vi "Illini Hyperloop GUI v3.1.vi"() -> ()   [LabVIEW 2015]
uses:
  <vilib>/robotics/Controls/Attitude Indicator/Attitude Indicator.xctl
  CommunicationStatus.ctl
  StageEnum.ctl
  BlockDiagramControlEnum.ctl
  <vilib>/ErrorRing/Error Ring.xnode
panel:
  out "Braking Force":dbl
  out "Braking Force Chart":dbl(slide) caption="Braking Force (N)" scale=0.0..10000.0
  out "Current 6":dbl[unit] caption="Current"
  out "Voltage 6":dbl[unit] caption="Voltage"
  out "RPM 6":dbl[unit] caption="RPM"
  out "Current 5":dbl[unit] caption="Current"
  out "Voltage 5":dbl[unit] caption="Voltage"
  out "RPM 5":dbl[unit] caption="RPM"
  out "Current 4":dbl[unit] caption="Current"
  out "Voltage 4":dbl[unit] caption="Voltage"
  out "RPM 4":dbl[unit] caption="RPM"
  out "Current 3":dbl[unit] caption="Current"
  out "Voltage 3":dbl[unit] caption="Voltage"
  out "RPM 3":dbl[unit] caption="RPM"
  out "Current 2":dbl[unit] caption="Current"
  out "Voltage 2":dbl[unit] caption="Voltage"
  out "RPM 2":dbl[unit] caption="RPM"
  out "Current 1":dbl[unit] caption="Current"
  out "Voltage 1":dbl[unit] caption="Voltage"
  out "RPM 1":dbl[unit] caption="RPM"
  out "Flight Time":string
  out "Attitude Indicator":cluster{"Roll":dbl, "Pitch":dbl}(xcontrol)
  out "Yaw":dbl(knob) scale=-20.0..20.0
  out "RPM Gauge 6":dbl(knob) scale=0.0..2000.0
  out "RPM Gauge 5":dbl(knob) scale=0.0..2000.0
  out "RPM Gauge 4":dbl(knob) scale=0.0..2000.0
  out "RPM Gauge 3":dbl(knob) scale=0.0..2000.0
  out "RPM Gauge 2":dbl(knob) scale=0.0..2000.0
  out "RPM Gauge 1":dbl(knob) scale=0.0..2000.0
  out "Cabin Pressure":dbl format="%#.3g"
  out "Cabin Pressure (psi)":dbl(graph)
  out "Stage":T1
  out "Communication Status":T2
  out "Levitation Height":dbl[unit]
  out "Computing:":dbl format="%#.2g"
  out "Low Battery":dbl format="%#.2g"
  out "High Battery:":dbl format="%#.2g"
  out "Battery 3":dbl(slide) scale=0.0..100.0
  out "Battery 2":dbl(slide) scale=0.0..100.0
  out "Battery 1":dbl(slide) scale=0.0..100.0
  out "Z acceleration":dbl
  out "Y acceleration":dbl
  out "X acceleration":dbl
  out "Z velocity":dbl
  out "Y velocity":dbl
  out "X velocity":dbl
  out "Z position":dbl
  out "Y position":dbl
  out "X position":dbl
  out "Position (m)":dbl(slide) scale=0.0..2490.0
  out "Checkmark":u16(ring)
  out "Velocity (m/s)":dbl(graph)
  in  "EMERGENCY BRAKE":bool
  in  "Functional Test Tab Control":T3(tab)
  out "Functional Test A Data":string caption="Data:"
  in  "Functional Test 1":bool caption="Boolean"
  out "Functional Test B Data":string caption="Data:"
  in  "Functional Test 2":bool caption="Boolean"
  out "Functional Test C Data":string caption="Data:"
  in  "Functional Test 3":bool caption="Boolean"
  in  "Functional Test 4":bool caption="Boolean"
  out "Functional Test D Data":string caption="Data:"
  in  "Client Closed":string="The client VI closed the connection."
  out "Data out":string
  out "remote address":string
  out "remote port":u16
  in  "Prepare for Launch":bool caption="Boolean"
  in  "Stop Program":bool
  out "Temp 2:":dbl format="%.2g"
  out "Temp 1:":dbl format="%.2g"
  out "Temperature (K)":dbl[](graph)
  out "Acceleration Chart":dbl(graph)
  # "Illini Hyperloop"
  # "Arx Pax"
  # "Front"
  # "Attitude"
  # "Acceleration (m/s/s)"
  # "Battery Levels (%)"
  # "More battery?????"
  # "Functional Test A: Power Up and Communication"
  # "Functional Test B: Levitation"
  # "Functional Test C: Communication Inside Tube"
  # "Functional Test D: Internal power and Levitation"
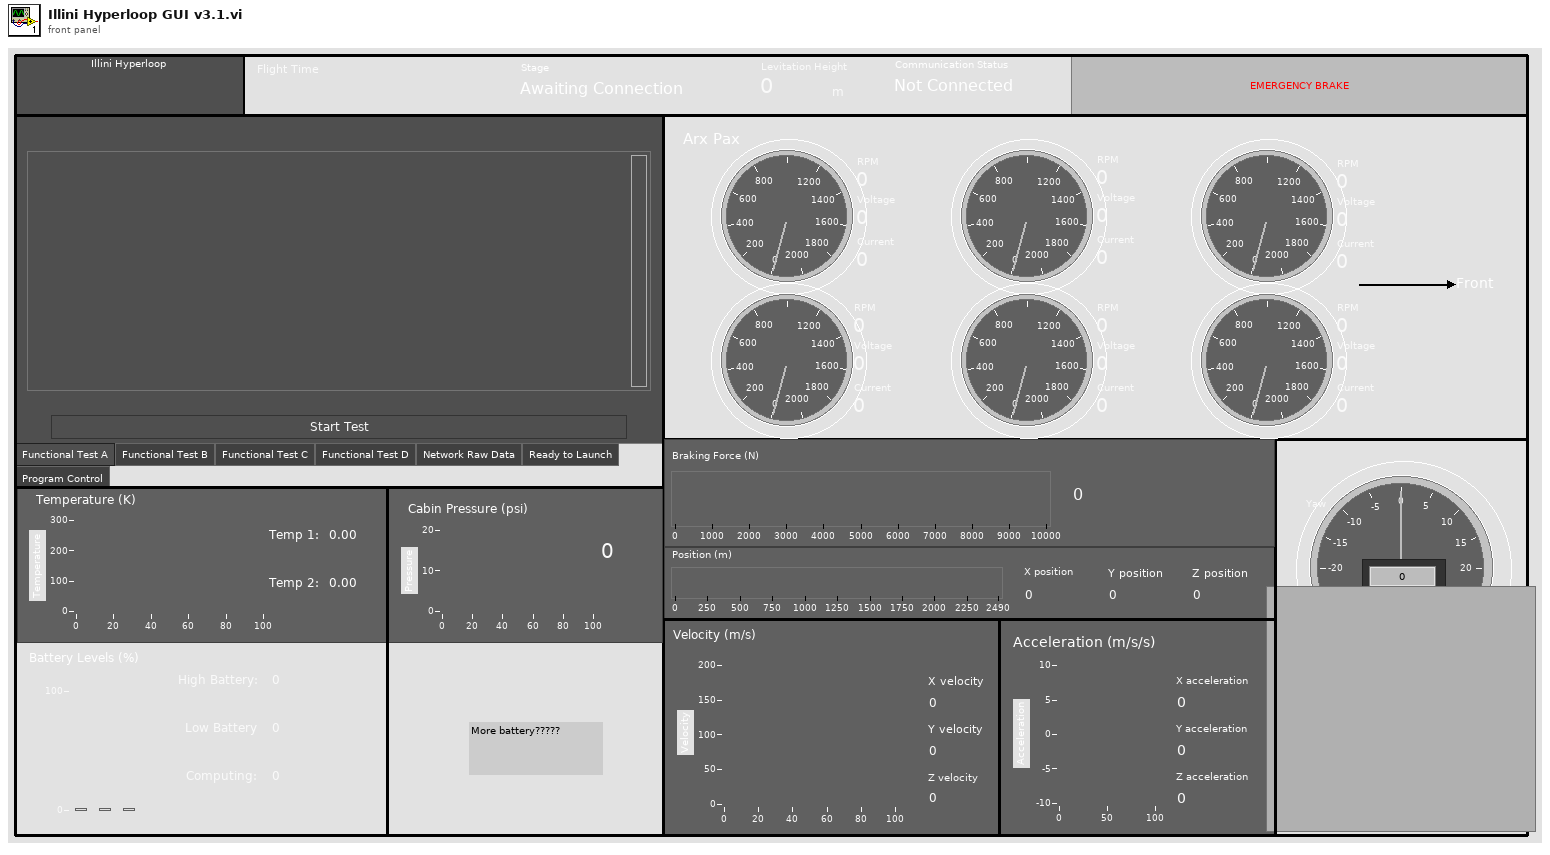
[diagram p1: front panel]
types:
  T1 = typedef "StageEnum.ctl" = enum16{"Awaiting Connection", "TEST Comms", "TEST Lev", "TEST Inside Comms", "TEST Internal Power", "Ready to Launch", "Acceleration", "Coast", "Brake"}
  T2 = typedef "CommunicationStatus.ctl" = enum16{"Not Connected", "Connected", "Disconnected"}
  T3 = enum32{"Functional Test A", "Functional Test B", "Functional Test C", "Functional Test D", "Network Raw Data", "Ready to Launch", "Program Control"}
  T4 = typedef "BlockDiagramControlEnum.ctl" = enum16{"Not Connected", "Disconnected", "Functional Test A", "Functional Test B", "Functional Test C", "Functional Test D", "Flight"}
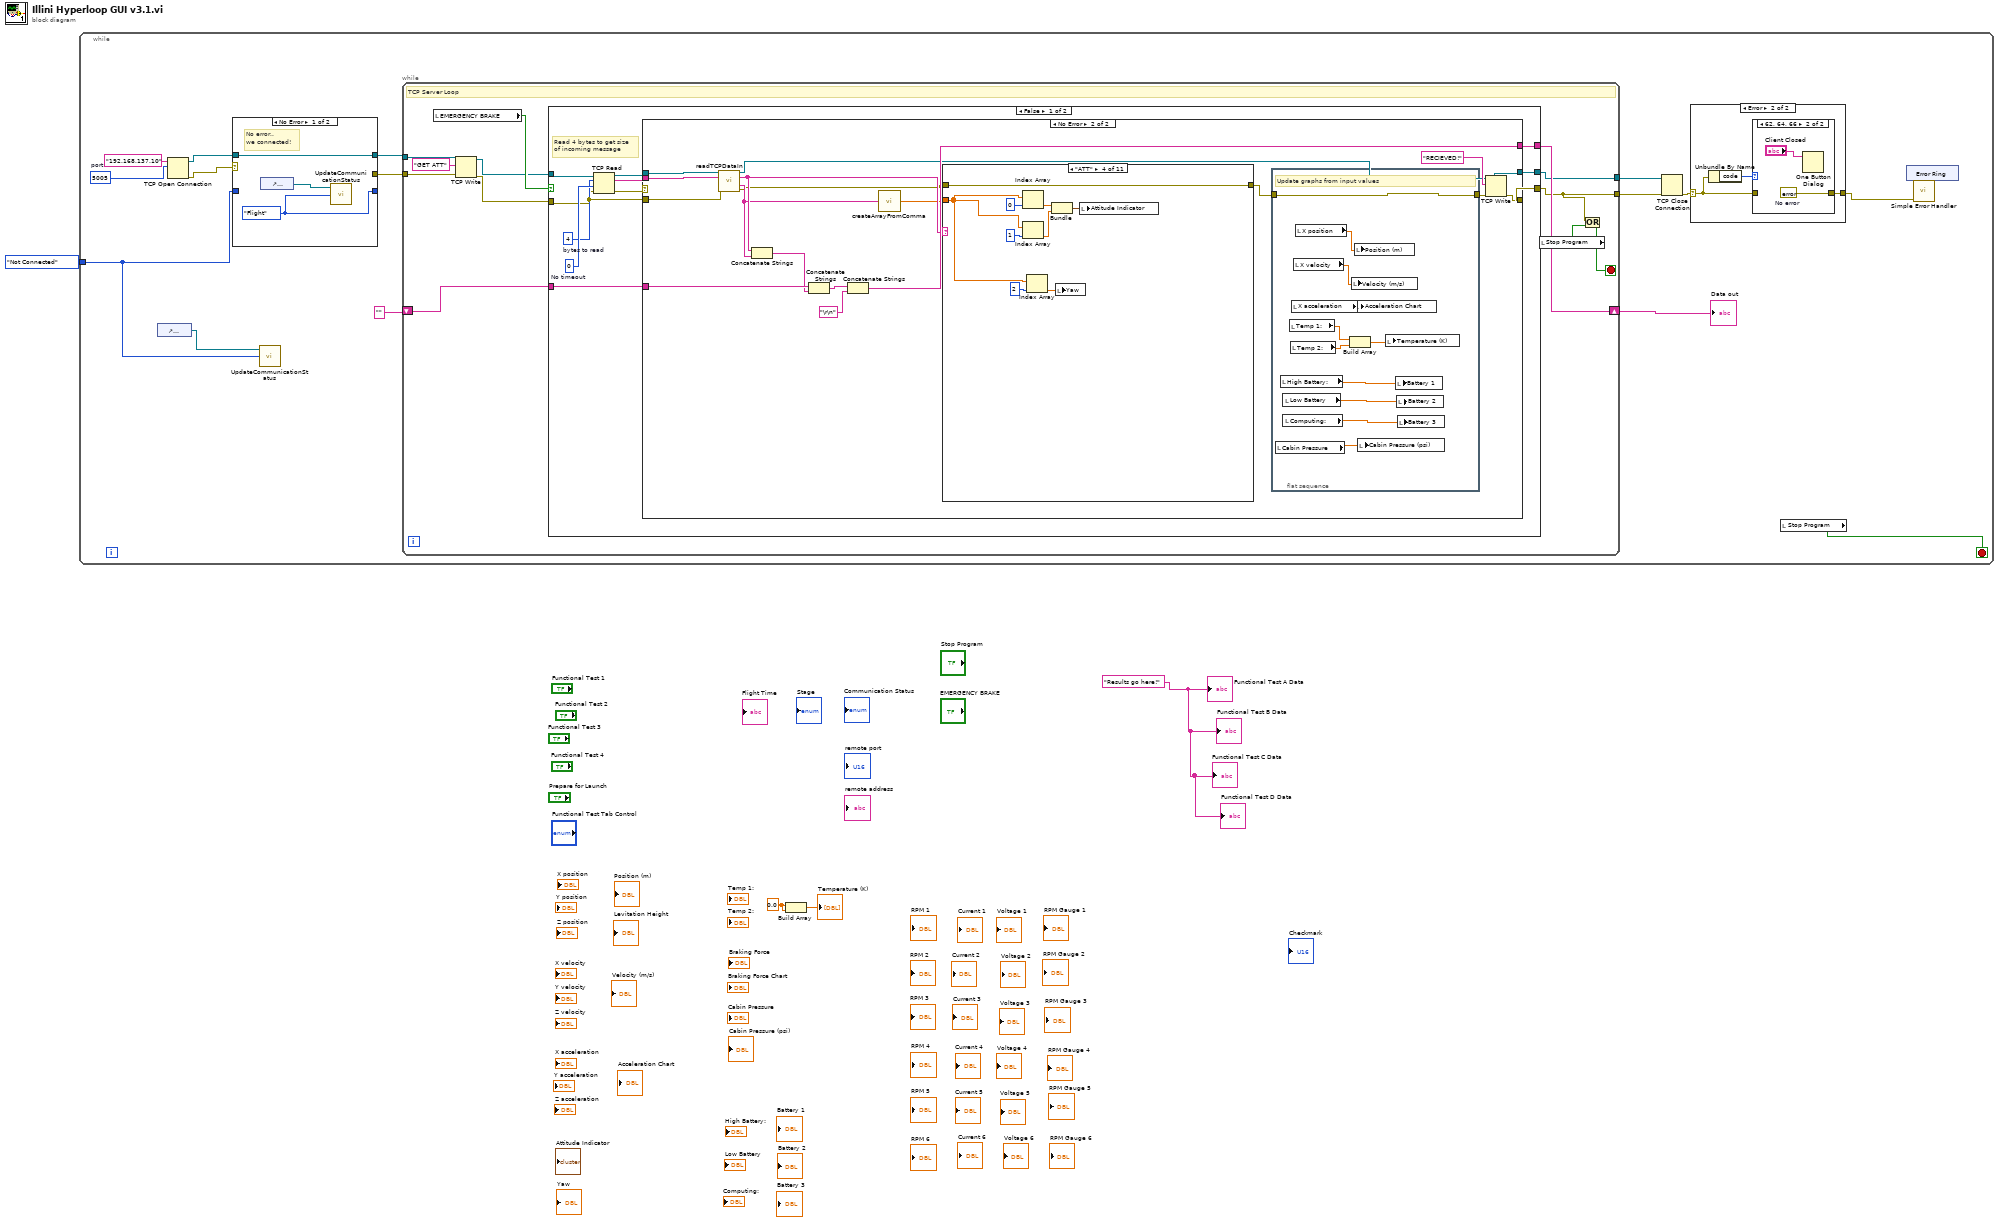
[diagram p0: block diagram]
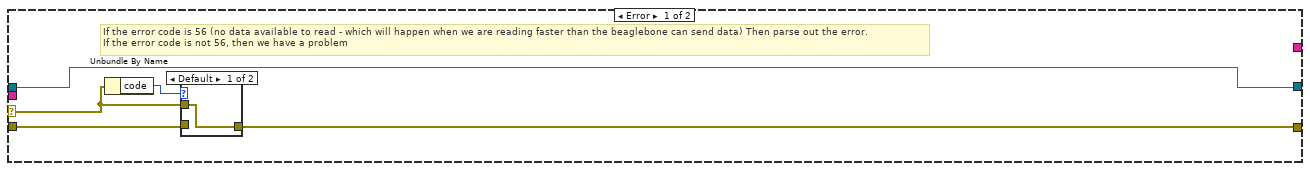
[diagram p5: hidden frame]
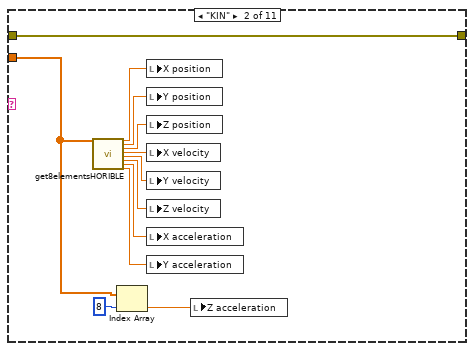
[diagram p8: hidden frame]
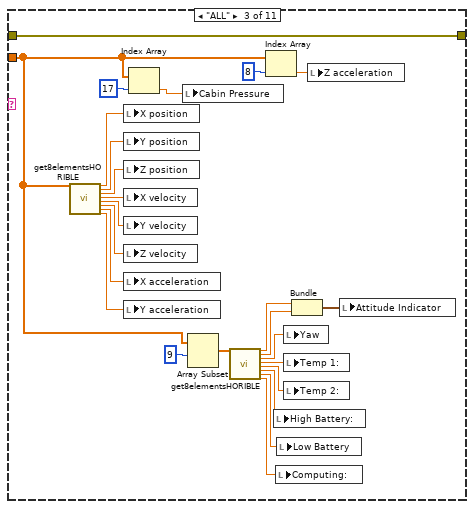
[diagram p9: hidden frame]
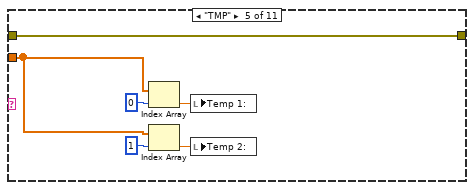
[diagram p10: hidden frame]
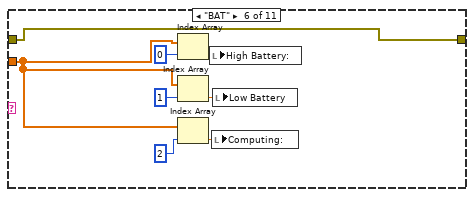
[diagram p11: hidden frame]
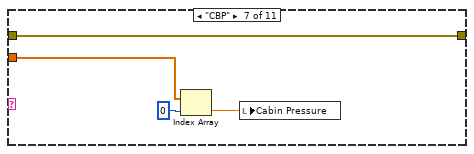
[diagram p12: hidden frame]
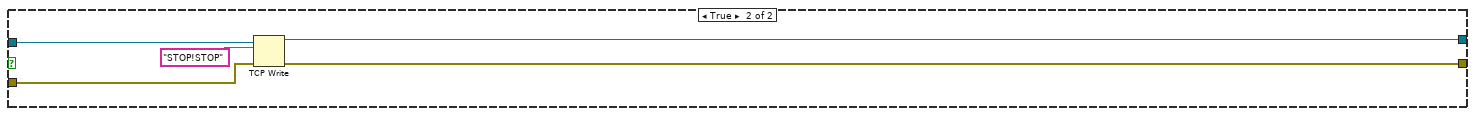
[diagram p17: hidden frame]
diagram:
  w2 = 0.0 ("element")
  w4 = "Results go here!" ("Functional Test 1 Data")
  n1 = while {
    tunnel: BlockDiagramControlEnum."Not Connected" -> [w9]
    stop <- w13 stop-if-true
    w8 = u16 5005  # port
    n2 = control-ref of="Communication Status"() -> (w10:refnum<vi>)
    n3 = TCP Open Connection(address="192.168.137.10", remote port or service name=w8) -> (connection ID=w6:refnum<k5>, error out=w7:errorcluster)  [unwired: 3 in]
    n4 = case shown="No Error" w7 {
      selector: w7 -> [_ w24]
      tunnel: w6 -> [w22 w25]
      tunnel: [w22 w25] -> w12
      tunnel: [_ w24] -> w11
      tunnel: w9 -> [_ w23]
      tunnel: [w20 w23] -> _
      frame No Error {
        w20 = BlockDiagramControlEnum."Flight"
        # "No error.. \nwe connected!"
        n5 = control-ref of="Communication Status"() -> (w21:refnum<vi>)
        n6 = call "UpdateCommunicationStatus.vi"("Block Diagram Control Enum"=w20, "Communication Enum Refnum in"=w21) -> ()  [unwired: 1 in]
      }
      frame Error {
      }
    }
    n7 = call "UpdateCommunicationStatus.vi"("Block Diagram Control Enum"=w9, "Communication Enum Refnum in"=w10) -> ()  [unwired: 1 in]
    n8 = while {
      tunnel: w12 -> [w38]
      tunnel: w11 -> [w36]
      shift-right: [w44] -> w16
      shift-left: "" -> [w45]
      tunnel: [w43] -> w15
      tunnel: [w40] -> w14
      stop <- w39 stop-if-true
      # "TCP Server Loop"
      n9 = local read "EMERGENCY BRAKE"() -> (w42:bool)
      n10 = TCP Write(connection ID=w38, data in="GET ATT", error in (no error)=w36) -> (connection ID out=w37:refnum<k5>, error out=w35:errorcluster)  [unwired: 1 in, 1 out]
      n11 = case shown="False" w42 {
        tunnel: w35 -> [w54 w166]
        tunnel: w37 -> [w55 w165]
        tunnel: [w50 w164] -> w43
        tunnel: [w52 w163] -> w40
        tunnel: w45 -> [w48 _]
        tunnel: [w47 _] -> w44
        frame False {
          w56 = 4  # bytes to read
          w57 = 0  # No timeout
          # "Read 4 bytes to get size\nof incoming message"
          n12 = TCP Read(connection ID=w55, bytes to read=w56, error in (no error)=w54, 9:w57) -> (connection ID out=w51:refnum<k5>, data out=w49:string, error out=w53:errorcluster)  [unwired: 1 in]
          n13 = case shown="No Error" w53 {
            selector: w53 -> [w60 _]
            tunnel: w54 -> [w61 w80]
            tunnel: [w59 w65] -> w52
            tunnel: w51 -> [w58 w81]
            tunnel: [w58 w67] -> w50
            tunnel: w49 -> [_ w82]
            tunnel: w48 -> [_ w79]
            tunnel: [_ w75] -> w47
            frame Error {
              # "If the error code is 56 (no data available to read - which will happen when we are reading faster than the beaglebone can send data) Then parse out the error. \nIf the error code is not 56, then we have a problem"
              n14 = Unbundle By Name(w60) -> ("code"=w62:i32)
              n15 = case shown="Default" w62 {
                tunnel: w60 -> [w63 _]
                tunnel: [w63 w64] -> w59
                tunnel: w61 -> [_ w64]
                frame Default {
                }
                frame 56 {
                }
              }
            }
            frame No Error {
              n16 = call "readTCPDataIn.vi"("TCP Network Connection in"=w81, "Size of data"=w82, "error in (no error)"=w80) -> ("TCP Network Connection out"=w68:refnum<k5>, "Operation"=w74:string, "Data"=w72:string, "error out"=w70:errorcluster)  [unwired: 8 in, 1 out]
              n17 = Concatenate Strings(w74, w72) -> (w73:string)
              n18 = Concatenate Strings(w79, w73) -> (w76:string)
              n19 = Concatenate Strings(w76, "\r\n") -> (w75:string)
              n20 = call "createArrayFromComma.vi"("String"=w72) -> ("Array"=w71:dbl[])
              n21 = case shown="\"ATT\"" w74 {
                tunnel: w71 -> [_ w105 w109 w137 w144 w151 w157 _ _ _ _]
                tunnel: w70 -> [w94 w103 w107 w132 w141 w147 w155 w159 w160 w161 w162]
                tunnel: [w94 w103 w107 w132 w141 w147 w155 w159 w160 w161 w162] -> w78
                frame Default {
                }
                frame "KIN" {
                  n22 = call "get8elementsHORIBLE.vi"("Array"=w105) -> ("Numeric"=w102:dbl, "Numeric 2"=w101:dbl, "Numeric 3"=w100:dbl, "Numeric 4"=w99:dbl, "Numeric 5"=w98:dbl, "Numeric 6"=w97:dbl, "Numeric 7"=w96:dbl, "Numeric 8"=w95:dbl)  [unwired: 19 in]
                  n23 = Index Array(array=w105, index=8) -> (element=w104:dbl)
                  n24 = local write "X position"(w102) -> ()
                  n25 = local write "Y position"(w101) -> ()
                  n26 = local write "Z position"(w100) -> ()
                  n27 = local write "X velocity"(w99) -> ()
                  n28 = local write "Y velocity"(w98) -> ()
                  n29 = local write "Z velocity"(w97) -> ()
                  n30 = local write "X acceleration"(w96) -> ()
                  n31 = local write "Y acceleration"(w95) -> ()
                  n32 = local write "Z acceleration"(w104) -> ()
                }
                frame "ALL" {
                  n33 = call "get8elementsHORIBLE.vi"("Array"=w109) -> ("Numeric"=w129:dbl, "Numeric 2"=w128:dbl, "Numeric 3"=w127:dbl, "Numeric 4"=w126:dbl, "Numeric 5"=w125:dbl, "Numeric 6"=w124:dbl, "Numeric 7"=w123:dbl, "Numeric 8"=w122:dbl)  [unwired: 19 in]
                  n34 = local write "X position"(w129) -> ()
                  n35 = local write "Y position"(w128) -> ()
                  n36 = local write "Z position"(w127) -> ()
                  n37 = local write "X velocity"(w126) -> ()
                  n38 = local write "Y velocity"(w125) -> ()
                  n39 = local write "Z velocity"(w124) -> ()
                  n40 = local write "X acceleration"(w123) -> ()
                  n41 = local write "Y acceleration"(w122) -> ()
                  n42 = Index Array(array=w109, index=17) -> (element=w108:dbl)
                  n43 = local write "Cabin Pressure"(w108) -> ()
                  n44 = Array Subset(array=w109, index=9) -> (w119:dbl[])  [unwired: 1 in]
                  n45 = call "get8elementsHORIBLE.vi"("Array"=w119) -> ("Numeric"=w118:dbl, "Numeric 2"=w117:dbl, "Numeric 3"=w116:dbl, "Numeric 4"=w115:dbl, "Numeric 5"=w114:dbl, "Numeric 6"=w113:dbl, "Numeric 7"=w112:dbl, "Numeric 8"=w111:dbl)  [unwired: 19 in]
                  n46 = Index Array(array=w109, index=8) -> (element=w130:dbl)
                  n47 = local write "High Battery:"(w113) -> ()
                  n48 = local write "Computing:"(w111) -> ()
                  n49 = local write "Low Battery"(w112) -> ()
                  n50 = local write "Yaw"(w116) -> ()
                  n51 = local write "Temp 1:"(w115) -> ()
                  n52 = local write "Temp 2:"(w114) -> ()
                  n53 = Bundle("Numeric"=w118, "Numeric 2"=w117) -> (w121:cluster{"Numeric":dbl, "Numeric 2":dbl})  [unwired: 1 in]
                  n54 = local write "Z acceleration"(w130) -> ()
                  n55 = local write "Attitude Indicator"(w121) -> ()
                }
                frame "ATT" {
                  n56 = Index Array(array=w137, index=0) -> (element=w136:dbl)
                  n57 = Index Array(array=w137, index=1) -> (element=w135:dbl)
                  n58 = Index Array(array=w137, index=2) -> (element=w133:dbl)
                  n59 = Bundle(w136, w135) -> (w134:cluster{dbl, dbl})  [unwired: 1 in]
                  n60 = local write "Yaw"(w133) -> ()
                  n61 = local write "Attitude Indicator"(w134) -> ()
                }
                frame "TMP" {
                  n62 = Index Array(array=w144, index=0) -> (element=w143:dbl)
                  n63 = Index Array(array=w144, index=1) -> (element=w142:dbl)
                  n64 = local write "Temp 1:"(w143) -> ()
                  n65 = local write "Temp 2:"(w142) -> ()
                }
                frame "BAT" {
                  n66 = Index Array(array=w151, index=0) -> (element=w150:dbl)
                  n67 = Index Array(array=w151, index=1) -> (element=w149:dbl)
                  n68 = Index Array(array=w151, index=2) -> (element=w148:dbl)
                  n69 = local write "High Battery:"(w150) -> ()
                  n70 = local write "Computing:"(w148) -> ()
                  n71 = local write "Low Battery"(w149) -> ()
                }
                frame "CBP" {
                  n72 = Index Array(array=w157, index=0) -> (element=w156:dbl)
                  n73 = local write "Cabin Pressure"(w156) -> ()
                }
                frame "FTA" {
                }
                frame "FTB" {
                }
                frame "FCC" {
                }
                frame "FCD" {
                }
              }
              n74 = flat-sequence {
                tunnel: w78 -> [w90]
                tunnel: [w90] -> w66
                frame #0 {
                  # "Update graphs from input values"
                  n75 = local read "Cabin Pressure"() -> (w86:dbl)
                  n76 = local read "High Battery:"() -> (w89:dbl)
                  n77 = local read "Low Battery"() -> (w88:dbl)
                  n78 = local read "Computing:"() -> (w87:dbl)
                  n79 = local read "Temp 1:"() -> (w85:dbl)
                  n80 = local read "Temp 2:"() -> (w84:dbl)
                  n81 = local read "X acceleration"() -> (w91:dbl)
                  n82 = local read "X velocity"() -> (w92:dbl)
                  n83 = local read "X position"() -> (w93:dbl)
                  n84 = Build Array(w85, w84) -> (w83:dbl[])
                  n85 = local write "Velocity (m/s)"(w92) -> ()
                  n86 = local write "Acceleration Chart"(w91) -> ()
                  n87 = local write "Position (m)"(w93) -> ()
                  n88 = local write "Cabin Pressure (psi)"(w86) -> ()
                  n89 = local write "Temperature (K)"(w83) -> ()
                  n90 = local write "Battery 1"(w89) -> ()
                  n91 = local write "Battery 2"(w88) -> ()
                  n92 = local write "Battery 3"(w87) -> ()
                }
              }
              n93 = TCP Write(connection ID=w68, data in="RECIEVED!", error in (no error)=w66) -> (connection ID out=w67:refnum<k5>, error out=w65:errorcluster)  [unwired: 1 in, 1 out]
            }
          }
        }
        frame True {
          n94 = TCP Write(connection ID=w165, data in="STOP!STOP", error in (no error)=w166) -> (connection ID out=w164:refnum<k5>, error out=w163:errorcluster)  [unwired: 1 in, 1 out]
        }
      }
      n95 = Wait (ms)(milliseconds to wait=u32 0) -> ()  [unwired: 1 out]
      n96 = local read "Stop Program"() -> (w41:bool)
      n97 = Or(x=w40, y=w41) -> (x .or. y?=w39:bool)
    }
    "Data out" <- w16
    n98 = TCP Close Connection(connection ID=w15, error in (no error)=w14) -> (error out=w19:errorcluster)  [unwired: 2 out]
    n99 = case shown="Error" w19 {
      selector: w19 -> [w27 w29]
      tunnel: [w27 w28] -> w18
      frame No Error {
      }
      frame Error {
        n100 = Unbundle By Name(w29) -> ("code"=w30:i32)
        n101 = case shown="62, 64, 66" w30 {
          tunnel: w29 -> [w31 _]
          tunnel: [w31 w33] -> w28
          frame Default {
          }
          frame 62, 64, 66 {
            w33 = errorcluster {"status"=FALSE, "code"=0, "source"=""}  # No error
            n102 = One Button Dialog(message="Client Closed") -> ()  [unwired: 1 in, 1 out]
          }
        }
      }
    }
    n103 = local read "Stop Program"() -> (w13:bool)
    n104 = xnode "Error Ring"() -> ()  [unwired: 1 out]
    n105 = call <vilib>:"Simple Error Handler.vi"("error in (no error)"=w18) -> ()  [unwired: 1 in, 8 out]
  }
  n106 = Build Array(w2, w2) -> (→"Temperature (K)":dbl[])
  "Functional Test A Data" <- w4
  "Functional Test B Data" <- w4
  "Functional Test C Data" <- w4
  "Functional Test D Data" <- w4
